vi "LED matrix.vi"   [LabVIEW 2018]
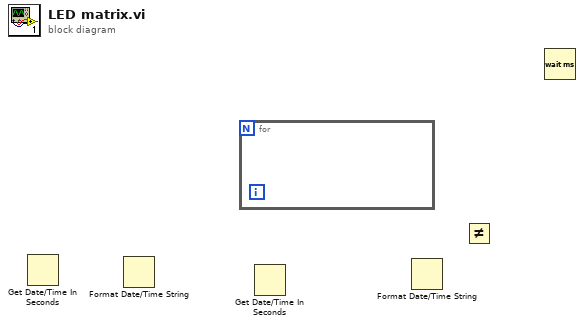
[diagram p0: block diagram]
diagram:
  n1 = Get Date/Time In Seconds() -> ()  [unwired: 1 out]
  n2 = Format Date/Time String() -> ()  [unwired: 3 in, 1 out]
  n3 = for {
  }
  n4 = Get Date/Time In Seconds() -> ()  [unwired: 1 out]
  n5 = Format Date/Time String() -> ()  [unwired: 3 in, 1 out]
  n6 = Not Equal?() -> ()  [unwired: 2 in, 1 out]
  n7 = Wait (ms)() -> ()  [unwired: 1 in, 1 out]
